vi "temp2.vi"() -> ()   [LabVIEW 2011]
panel:
  out "output cluster":cluster{dbl[], dbl[]}[](graph)
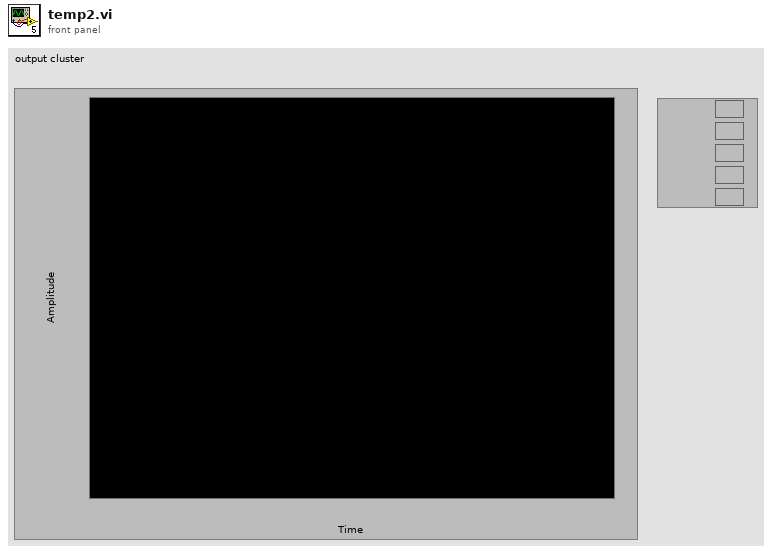
[diagram p1: front panel]
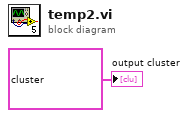
[diagram p0: block diagram]
diagram:
  "output cluster" <- cluster{dbl[], dbl[]}[] [{array[1266 elements], array[1266 elements]}, {array[1266 elements], array[1266 elements]}, {array[1266 elements], array[1266 elements]}, {array[1266 elements], array[1266 elements]}, {array[1266 elements], array[1266 elements]}] ("output cluster")
